vi "AlignTopBottom.vi"(6 "Variant in":variant, 7 "Shift Pressed?":bool, 8 "error in (no error)":errorcluster, 10 "QD Combo Box Ref":refnum<vi>, 11 "QD Launch VI Ref":refnum<vi>) -> (0 "error out":errorcluster, 4 "Variant out":variant)   [LabVIEW 2017]
doc: "Aligns top or bot. To align top press Ctrl+Shift+z\n\nDefault Shortcut - [$z]"
panel:
  in  "Undo Name":string="Quick Drop Keyboard Shortcut"
  # "Do not change the connector pane of this VI.\n\nSee the block diagram for directions on how to use this template."
  # "Specify the name of the Undo transaction"
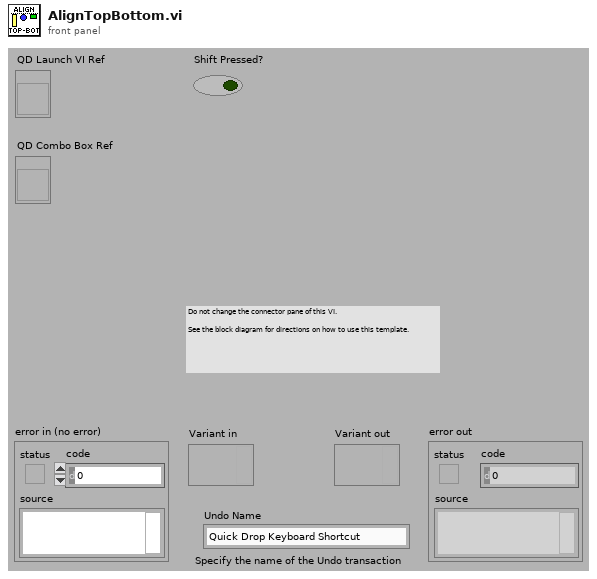
[diagram p1: front panel]
types:
  T1 = enum32{"Top Edges", "Vertical Centers", "Bottom Edges", "Left Edges", "Horizontal Centers", "Right Edges"}
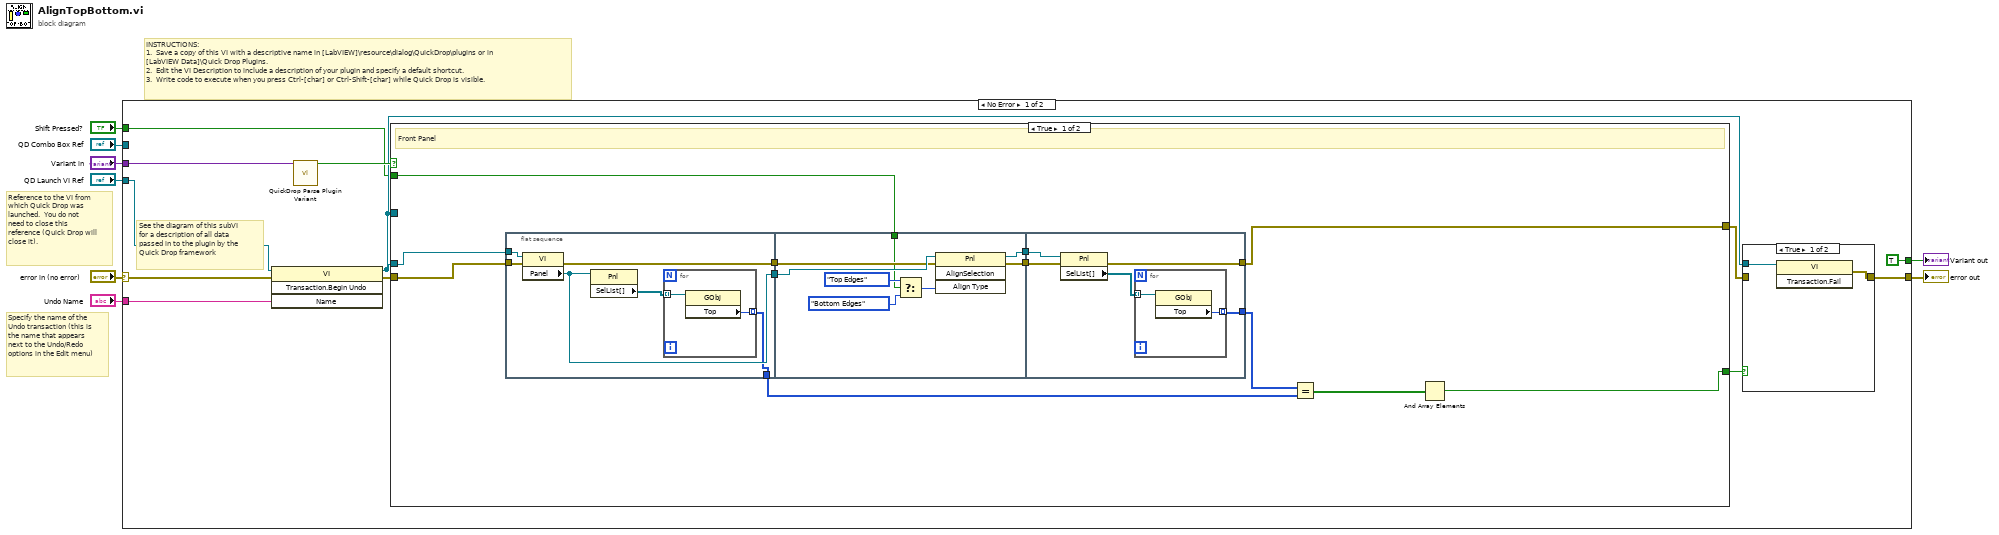
[diagram p0: block diagram]
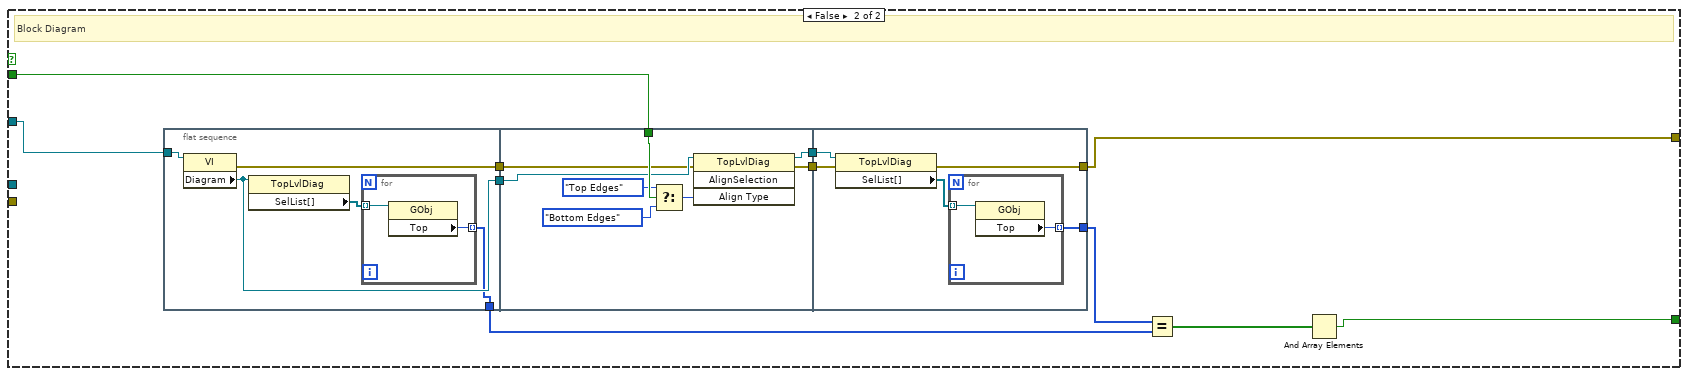
[diagram p2: hidden frame]
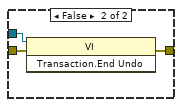
[diagram p3: hidden frame]
diagram:
  # "Specify the name of the Undo transaction (this is the name that appears next to the Undo/Redo options in the Edit menu)"
  # "Reference to the VI from which Quick Drop was launched.  You do not need to close this reference (Quick Drop will close it)."
  # "INSTRUCTIONS:\n1.  Save a copy of this VI with a descriptive name in [LabVIEW]\\resource\\dialog\\QuickDrop\\plugins or in [LabVIEW Data]\\Quick Drop Plugins.\n2.  Edit the VI Description to include a description of your plugin and specify a default shortcut. \n3.  Write code to execute when you press Ctrl-[char] or Ctrl-Shift-[char] while Quick Drop is visible."
  n1 = case shown="No Error" "error in (no error)" {
    selector: "error in (no error)" -> [w19 w94]
    tunnel: [w14 w94] -> w7
    tunnel: "QD Launch VI Ref" -> [w18 _]
    tunnel: "Shift Pressed?" -> [w11 _]
    tunnel: "QD Combo Box Ref" -> [_ _]
    tunnel: "Variant in" -> [w20 _]
    tunnel: "Undo Name" -> [w17 _]
    tunnel: [TRUE _] -> w1
    frame No Error {
      # "See the diagram of this subVI for a description of all data passed in to the plugin by the Quick Drop framework"
      n2 = invoke class="VI" method="Transaction.Begin Undo"(reference=w18, error in=w19, "Name"=w17) -> (reference out=w13:refnum<vi>, error out=w12:errorcluster)  [unwired: 1 in, 2 out]
      n3 = call <vilib>:"QuickDrop Parse Plugin Variant.vi"("QDKS Variant in"=w20) -> ("QD Launch VI Panel?"=w15:bool)  [unwired: 12 in, 2 out]
      n4 = case shown="True" w15 {
        tunnel: w12 -> [w24 _]
        tunnel: w13 -> [w25 _]
        tunnel: w13 -> [_ w66]
        tunnel: w11 -> [w21 w65]
        tunnel: [w22 w62] -> w10
        tunnel: [w23 w59] -> w9
        frame True {
          # "Front Panel"
          n5 = flat-sequence {
            tunnel: w25 -> [w38]
            tunnel: w24 -> [w37]
            tunnel: [w36] -> w32
            tunnel: [w35] -> w31
            tunnel: [w33] -> w27
            tunnel: w32 -> [w45]
            tunnel: w31 -> [w44]
            tunnel: [w43] -> w30
            tunnel: [w42] -> w29
            tunnel: w21 -> [w41]
            tunnel: [w52] -> w22
            tunnel: w30 -> [w53]
            tunnel: w29 -> [w51]
            tunnel: [w49] -> w28
            frame #0 {
              n6 = property class="VI"(reference=w38, error in=w37) -> (error out=w35:errorcluster, "Panel"=w36:refnum<vi>)  [unwired: 1 out]
              n7 = property class="Pnl"(reference=w36) -> ("SelList[]"=w34:refnum<vi>[])  [unwired: 1 in, 2 out]
              n8 = for {
                tunnel: [w40] -> w33 mode=indexing
                tunnel: w34 -> [w39] mode=indexing
                n9 = property class="GObj"(reference=w39) -> ("Top"=w40:i32)  [unwired: 1 in, 2 out]
              }
            }
            frame #1 {
              n10 = Select(t=T1."Top Edges" ("Align Type"), s=w41, f=T1."Bottom Edges" ("Align Type")) -> (s? t:f=w48:T1)
              n11 = invoke class="Pnl" method="AlignSelection"(reference=w45, error in=w44, "Align Type"=w48) -> (reference out=w42:refnum<vi>, error out=w43:errorcluster)  [unwired: 1 in, 2 out]
            }
            frame #2 {
              n12 = property class="Pnl"(reference=w51, error in=w53) -> (error out=w52:errorcluster, "SelList[]"=w50:refnum<vi>[])  [unwired: 1 out]
              n13 = for {
                tunnel: [w54] -> w49 mode=indexing
                tunnel: w50 -> [w55] mode=indexing
                n14 = property class="GObj"(reference=w55) -> ("Top"=w54:i32)  [unwired: 1 in, 2 out]
              }
            }
          }
          n15 = Equal?(x=w28, y=w27) -> (x = y?=w26:bool[])
          n16 = And Array Elements(Boolean array=w26) -> (logical AND=w23:bool)
        }
        frame False {
          # "Block Diagram"
          n17 = flat-sequence {
            tunnel: w66 -> [w71]
            tunnel: [w70] -> w64
            tunnel: [w69] -> w63
            tunnel: [w67] -> w57
            tunnel: w65 -> [w79]
            tunnel: w64 -> [w77]
            tunnel: w63 -> [w76]
            tunnel: [w75] -> w61
            tunnel: [w74] -> w60
            tunnel: [w85] -> w62
            tunnel: w61 -> [w86]
            tunnel: w60 -> [w84]
            tunnel: [w82] -> w58
            frame #0 {
              n18 = property class="VI"(reference=w71) -> (error out=w69:errorcluster, "Diagram"=w70:refnum<vi>)  [unwired: 1 in, 1 out]
              n19 = property class="TopLvlDiag"(reference=w70) -> ("SelList[]"=w68:refnum<vi>[])  [unwired: 1 in, 2 out]
              n20 = for {
                tunnel: [w73] -> w67 mode=indexing
                tunnel: w68 -> [w72] mode=indexing
                n21 = property class="GObj"(reference=w72) -> ("Top"=w73:i32)  [unwired: 1 in, 2 out]
              }
            }
            frame #1 {
              n22 = Select(t=T1."Top Edges" ("Align Type"), s=w79, f=T1."Bottom Edges" ("Align Type")) -> (s? t:f=w81:T1)
              n23 = invoke class="TopLvlDiag" method="AlignSelection"(reference=w77, error in=w76, "Align Type"=w81) -> (reference out=w74:refnum<vi>, error out=w75:errorcluster)  [unwired: 1 in, 2 out]
            }
            frame #2 {
              n24 = property class="TopLvlDiag"(reference=w84, error in=w86) -> (error out=w85:errorcluster, "SelList[]"=w83:refnum<vi>[])  [unwired: 1 out]
              n25 = for {
                tunnel: [w87] -> w82 mode=indexing
                tunnel: w83 -> [w88] mode=indexing
                n26 = property class="GObj"(reference=w88) -> ("Top"=w87:i32)  [unwired: 1 in, 2 out]
              }
            }
          }
          n27 = Equal?(x=w58, y=w57) -> (x = y?=w56:bool[])
          n28 = And Array Elements(Boolean array=w56) -> (logical AND=w59:bool)
        }
      }
      n29 = case shown="True" w9 {
        tunnel: w13 -> [w89 w92]
        tunnel: [w90 w93] -> w14
        tunnel: w10 -> [_ w91]
        frame True {
          n30 = invoke class="VI" method="Transaction.Fail"(reference=w89) -> (error out=w90:errorcluster)  [unwired: 2 in, 2 out]
        }
        frame False {
          n31 = invoke class="VI" method="Transaction.End Undo"(reference=w92, error in=w91) -> (error out=w93:errorcluster)  [unwired: 1 in, 2 out]
        }
      }
    }
    frame Error {
    }
  }
  "error out" <- w7
  "Variant out" <- w1
